vi "apply modification.vi"(10 "vis":refnum<vi>[](array[refnum]), 11 "cosmetic changes in":refnum<class "cosmetic changes.lvclass">) -> (0 "error report":errorcluster[](array[cluster]), 3 "cosmetic changes out":refnum<class "cosmetic changes.lvclass">)   [LabVIEW 2013, in "cosmetic changes.lvclass"]
uses:
  cosmetic changes.lvclass
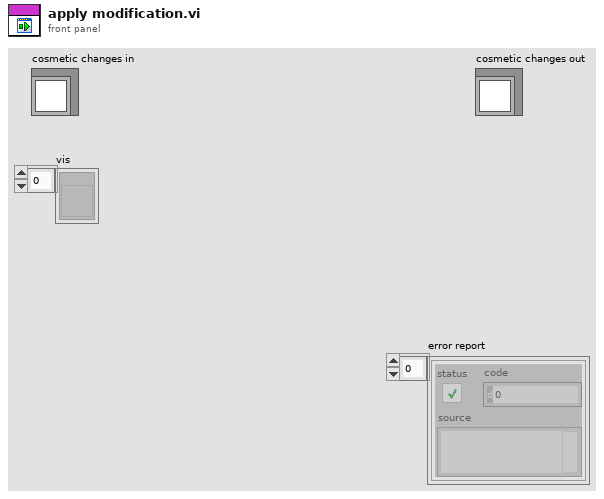
[diagram p1: front panel]
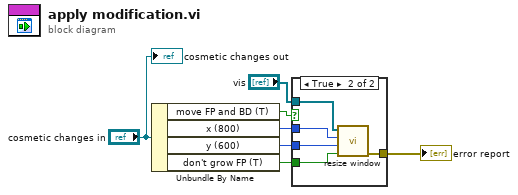
[diagram p0: block diagram]
diagram:
  n1 = Unbundle By Name("cosmetic changes in") -> ("move FP and BD (T)"=w6:bool, "x (800)"=w5:i16, "y (600)"=w4:i16, "don't grow FP (T)"=w3:bool)
  n2 = case shown="True" w6 {
    tunnel: "vis" -> [_ w12]
    tunnel: w5 -> [_ w11]
    tunnel: w4 -> [_ w10]
    tunnel: w3 -> [_ w9]
    tunnel: [_ w8] -> w2
    frame False {
    }
    frame True {
      n3 = call "resize window.vi"("don't grow front panels"=w9, "y (600)"=w10, "x (800)"=w11, "vis"=w12) -> ("error report"=w8:errorcluster[])  [unwired: 7 in]
    }
  }
  "error report" <- w2
  "cosmetic changes out" <- "cosmetic changes in"
